vi "Stepper Motor 2.3 Working.vi"() -> ()   [LabVIEW 2017]
uses:
  <vilib>/myRIO/Instrument Drivers/Onboard IO/DIO/typedefs/DIO Reference.ctl
  <vilib>/myRIO/Common/Instrument Driver Framework/Utilities/typedefs/myRIO Generic Hardware Reference.ctl
  <vilib>/myRIO/Common/Instrument Driver Framework/Utilities/typedefs/Hardware Version Enum.ctl
  <vilib>/myRIO/Common/Instrument Driver Framework/Utilities/typedefs/myRIO v1.0 Reference.ctl
  <vilib>/myRIO/Common/Instrument Driver Framework/Utilities/typedefs/Generic FPGA Reference.ctl
  <vilib>/myRIO/Common/Instrument Driver Framework/myRIO v1.0/DIO/typedefs/DIO Channels List.ctl
  <vilib>/myRIO/Common/Instrument Driver Framework/myRIO v1.0/DIO/typedefs/DIO Channels Enum.ctl
  <vilib>/userdefined/High Color/nirio_resource_hc.ctl
  <vilib>/myRIO/Common/Instrument Driver Framework/Utilities/vis/Is FPGA Ref Available.vi
  <vilib>/myRIO/Common/Instrument Driver Framework/myRIO v1.0/DIO/vis/myRIO v1.1 Open DIO.vi
  <vilib>/myRIO/Instrument Drivers/Onboard IO/DIO/vis/Write.vi
  <vilib>/myRIO/Common/Instrument Driver Framework/Utilities/vis/Validate Channels.vi
  <vilib>/myRIO/Common/Instrument Driver Framework/myRIO v1.0/DIO/vis/myRIO v1.0 Reserve DIO.vi
  <vilib>/myRIO/Common/Instrument Driver Framework/myRIO v1.0/Resource Manager/vis/myRIO v1.0 Reserve Channel List.vi
  <vilib>/myRIO/Common/Instrument Driver Framework/myRIO v1.0/DIO/vis/myRIO v1.0 Build MUX Configuration DIO.vi
  <vilib>/myRIO/Common/Instrument Driver Framework/myRIO v1.0/Resource Manager/vis/myRIO v1.0 Reserve Channel.vi
  <vilib>/myRIO/Common/Instrument Driver Framework/myRIO v1.0/Resource Manager/vis/myRIO v1.0 Unreserve Channel.vi
  <vilib>/myRIO/Common/Instrument Driver Framework/myRIO v1.0/Resource Manager/vis/myRIO v1.0 Create Configuration List.vi
  <vilib>/myRIO/Common/Instrument Driver Framework/myRIO v1.0/Resource Manager/vis/myRIO v1.0 Build Mutex Name.vi
  <vilib>/Utility/VariantDataType/GetNumericInfo.vi
  <vilib>/Utility/error.llb/Error Cluster From Error Code.vi
  <vilib>/myRIO/Common/Instrument Driver Framework/myRIO v1.0/myRIO v1.1 Open.vi
  <vilib>/myRIO/Common/Instrument Driver Framework/Utilities/vis/IO Manager.vi
  <vilib>/myRIO/Common/Instrument Driver Framework/Utilities/vis/Configuration Manager.vi
  <vilib>/myRIO/Common/Instrument Driver Framework/myRIO v1.0/Resource Manager/vis/myRIO v1.0 Configure IO.vi
  <vilib>/myRIO/Common/Instrument Driver Framework/myRIO v1.0/myRIO v1.0 Close.vi
  <vilib>/myRIO/Common/Instrument Driver Framework/myRIO v1.0/DIO/vis/myRIO v1.0 Write DIO.vi
  <vilib>/myRIO/Express VI/Onboard Devices/LED/LED Express VI.xnode
  <vilib>/myRIO/Instrument Drivers/Onboard IO/DIO/vis/myRIO DIO Open.xnode
  <vilib>/myRIO/Express VI/Onboard IO/DO/DO Express VI.xnode
  <vilib>/myRIO/Instrument Drivers/Onboard IO/DIO/DIO.lvlib
panel:
  in  "y (inches)":dbl
  out "current pps d":dbl
  out "loop num d":i32
  out "nc":dbl format="%.2f"
  out "current pps c":dbl
  out "loop num c":i32
  out "na":dbl format="%.2f"
  out "current pps a":dbl
  out "loop num a":i32
  in  "Dir":bool=TRUE
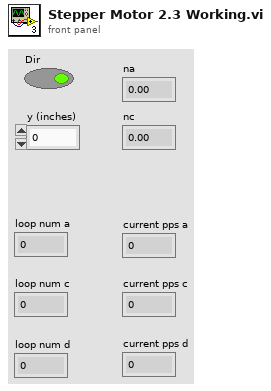
[diagram p1: front panel]
types:
  T1 = typedef "DIO.lvlib/DIO Reference.ctl" = cluster{"myRIO Reference":T2, "DIO Channels List":T6}
  T2 = typedef "myRIO Generic Hardware Reference.ctl" = cluster{"myRIO Model":T3, "myRIO Hardware Reference":T4}
  T3 = typedef "Hardware Version Enum.ctl" = enum16{"Unknown", "myRIO-1900", "myRIO-1950", "roboRIO", "NI ELVIS RIO CM"}
  T4 = typedef "myRIO v1.0 Reference.ctl" = cluster{"Generic FPGA Reference":T5, "Allow multiple opens":bool}
  T5 = typedef "Generic FPGA Reference.ctl" = refnum<k20>
  T6 = typedef "DIO Channels List.ctl" = T7[]
  T7 = typedef "DIO Channels Enum.ctl" = enum16{"Not Connected", "C/DIO0", "C/DIO1", "C/DIO2", "C/DIO3", "C/DIO4", "C/DIO5", "C/DIO6", "C/DIO7", "A/DIO0", "A/DIO1", "A/DIO2", "A/DIO3", "A/DIO4", "A/DIO5", "A/DIO6", "A/DIO7", "A/DIO8", "A/DIO9", "A/DIO10", "A/DIO11", "A/DIO12", "A/DIO13", "A/DIO14", "A/DIO15", "B/DIO0", "B/DIO1", "B/DIO2", "B/DIO3", "B/DIO4", "B/DIO5", "B/DIO6", "B/DIO7", "B/DIO8", "B/DIO9", "B/DIO10", "B/DIO11", "B/DIO12", "B/DIO13", "B/DIO14", "B/DIO15", "LED0", "LED1", "LED2", "LED3", "Button0", "DIO/DIO0", "DIO/DIO1", "DIO/DIO2", "DIO/DIO3", "DIO/DIO4", "DIO/DIO5", "DIO/DIO6", "DIO/DIO7", "DIO/DIO8", "DIO/DIO9", "SPI/CS0", "SPI/CS1", "SPI/CS2", "SPI/CS3", "LED RADIO (Green)", "LED RADIO (Red)", "LED COMM (Green)", "LED COMM (Red)", "LED MODE (Green)", "LED MODE (Red)"}
  T8 = typedef "nirio_resource_hc.ctl" = tag
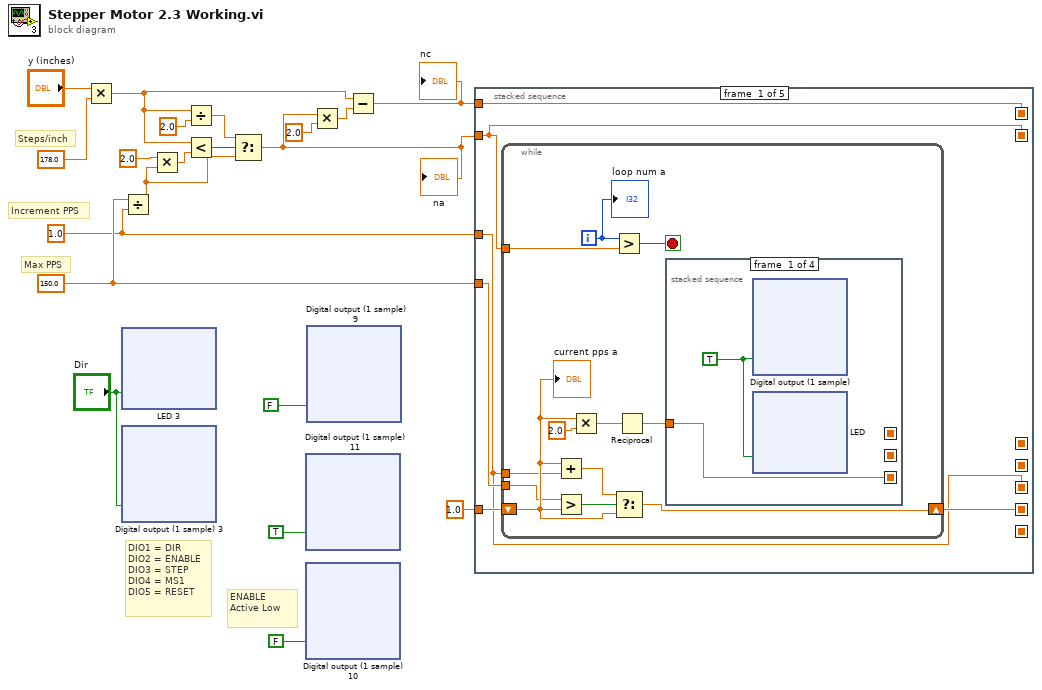
[diagram p0: block diagram]
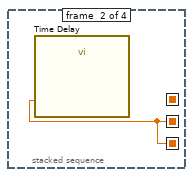
[diagram p2: hidden frame]
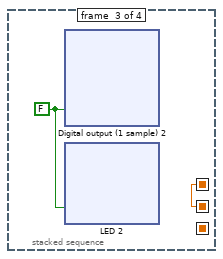
[diagram p3: hidden frame]
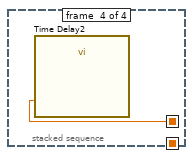
[diagram p4: hidden frame]
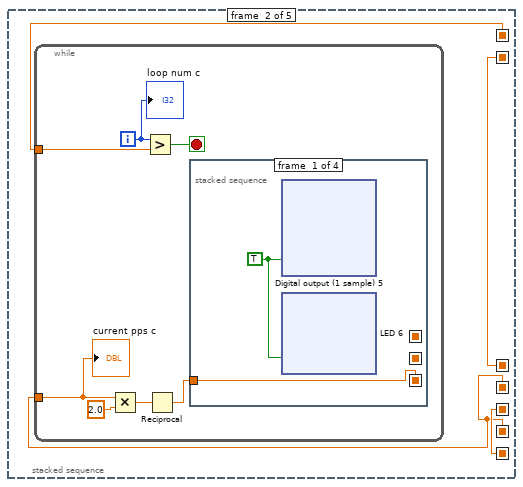
[diagram p5: hidden frame]
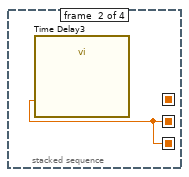
[diagram p6: hidden frame]
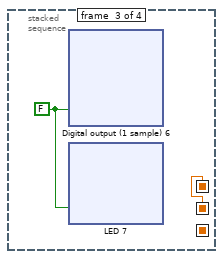
[diagram p7: hidden frame]
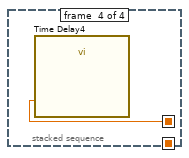
[diagram p8: hidden frame]
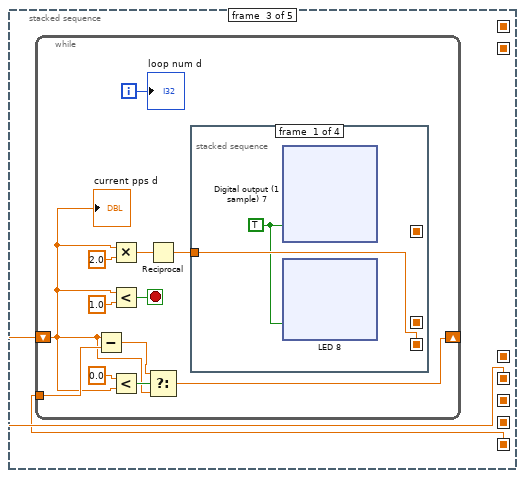
[diagram p9: hidden frame]
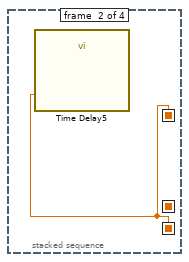
[diagram p10: hidden frame]
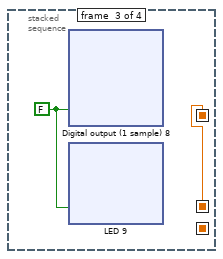
[diagram p11: hidden frame]
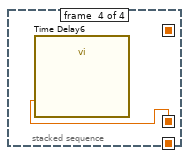
[diagram p12: hidden frame]
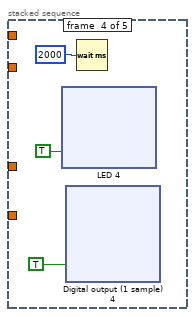
[diagram p13: hidden frame]
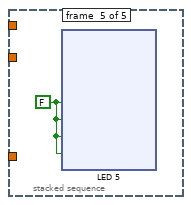
[diagram p14: hidden frame]
diagram:
  w15 = 1.0 ("increment pps")
  w16 = 150.0 ("max pps")
  # "Increment PPS"
  # "Steps/inch"
  # "Max PPS"
  # "ENABLE\nActive Low"
  # "DIO1 = DIR\nDIO2 = ENABLE\nDIO3 = STEP\nDIO4 = MS1\nDIO5 = RESET"
  n1 = Multiply(x="y (inches)", y=178.0 ("steps/in")) -> (x*y=w7:dbl)
  n2 = xnode "LED 3"("LED0"="Dir") -> ()  [unwired: 1 in, 1 out]
  n3 = xnode "Digital output (1 sample) 3"("DIR (A/DIO1 (Pin 13))"="Dir") -> ()  [unwired: 1 in, 1 out]
  n4 = Divide(x=w16, y=w15) -> (x/y=w4:dbl)
  n5 = Multiply(x=2.0 ("y"), y=w4) -> (x*y=w14:dbl)
  n6 = Divide(x=w7, y=2.0) -> (x/y=w11:dbl)
  n7 = Less?(x=w7, y=w14) -> (x < y?=w13:bool)
  n8 = Select(t=w11, s=w13, f=w4) -> (s? t:f=w8:dbl)
  "na" <- w8
  n9 = xnode "Digital output (1 sample) 11"("A/DIO5 (Pin 21)"=TRUE) -> ()  [unwired: 1 in, 1 out]
  n10 = xnode "Digital output (1 sample) 10"("A/DIO2 (Pin 15)"=FALSE) -> ()  [unwired: 1 in, 1 out]
  n11 = xnode "Digital output (1 sample) 9"("A/DIO4 (Pin 19)"=FALSE) -> ()  [unwired: 1 in, 1 out]
  n12 = Multiply(x=w8, y=2.0) -> (x*y=w10:dbl)
  n13 = Subtract(x=w7, y=w10) -> (x-y=w6:dbl)
  "nc" <- w6
  n14 = stacked-sequence {
    seq-local: [w24 _ _ _ _] -> [_ w185 _ _ _]
    seq-local: [w23 _ _ _ _] -> [_ w186 _ _ _]
    seq-local: [w22 _ _ _ _] -> [_ w188 _ _ _]
    seq-local: [w21 _ _ _ _] -> [_ w187 _ _ _]
    seq-local: [_ w188 _ _ _] -> [_ _ w342 _ _]
    seq-local: [_ w187 _ _ _] -> [_ _ _ _ _]
    seq-local: [_ w186 _ _ _] -> [_ _ w343 _ _]
    tunnel: w16 -> [w26 _ _ _ _]
    tunnel: w15 -> [w22 _ _ _ _]
    tunnel: 1.0 ("starting pps") -> [w25 _ _ _ _]
    tunnel: w8 -> [w21 _ _ _ _]
    tunnel: w6 -> [w24 _ _ _ _]
    frame #0 {
      n15 = while {
        shift-right: [w33] -> w23
        shift-left: w25 -> [w32]
        tunnel: w26 -> [w31]
        tunnel: w22 -> [w30]
        tunnel: w21 -> [w28]
        i -> [w27]
        stop <- w29 stop-if-true
        n16 = Add(x=w32, y=w30) -> (x+y=w34:dbl)
        n17 = Greater?(x=w31, y=w32) -> (0:w35:bool)
        n18 = Multiply(x=w32, y=2.0) -> (x*y=w38:dbl)
        n19 = Greater?(x=w27, y=w28) -> (0:w29:bool)
        n20 = Select(t=w34, s=w35, f=w32) -> (s? t:f=w33:dbl)
        n21 = Reciprocal(x=w38) -> (1/x=w36:dbl)
        n22 = stacked-sequence {
          seq-local: [w40 _ _ _] -> [_ w111 _ _]
          seq-local: [_ w111 _ _] -> [_ _ w113 _]
          seq-local: [_ _ w113 _] -> [_ _ _ w184]
          tunnel: w36 -> [w40 _ _ _]
          frame #0 {
            w39 = TRUE
            n23 = xnode "Digital output (1 sample)"("A/DIO3 (Pin 17)"=w39) -> ()  [unwired: 1 in, 1 out]
            n24 = xnode "LED"("LED1"=w39) -> ()  [unwired: 1 in, 1 out]
          }
          frame #1 {
            n25 = call "Time Delay"("Delay Time (s)"=w111) -> ()  [unwired: 10 in, 1 out]
          }
          frame #2 {
            w112 = FALSE
            n26 = xnode "Digital output (1 sample) 2"("A/DIO3 (Pin 17)"=w112) -> ()  [unwired: 1 in, 1 out]
            n27 = xnode "LED 2"("LED1"=w112) -> ()  [unwired: 1 in, 1 out]
          }
          frame #3 {
            n28 = call "Time Delay2"("Delay Time (s)"=w184) -> ()  [unwired: 10 in, 1 out]
          }
        }
        "current pps a" <- w32
        "loop num a" <- w27
      }
    }
    frame #1 {
      n29 = while {
        tunnel: w185 -> [w190]
        tunnel: w186 -> [w192]
        i -> [w189]
        stop <- w191 stop-if-true
        n30 = Multiply(x=w192, y=2.0) -> (x*y=w195:dbl)
        n31 = Greater?(x=w189, y=w190) -> (0:w191:bool)
        n32 = Reciprocal(x=w195) -> (1/x=w193:dbl)
        n33 = stacked-sequence {
          seq-local: [w197 _ _ _] -> [_ w268 _ _]
          seq-local: [_ w268 _ _] -> [_ _ w270 _]
          seq-local: [_ _ w270 _] -> [_ _ _ w341]
          tunnel: w193 -> [w197 _ _ _]
          frame #0 {
            w196 = TRUE
            n34 = xnode "Digital output (1 sample) 5"("A/DIO3 (Pin 17)"=w196) -> ()  [unwired: 1 in, 1 out]
            n35 = xnode "LED 6"("LED1"=w196) -> ()  [unwired: 1 in, 1 out]
          }
          frame #1 {
            n36 = call "Time Delay3"("Delay Time (s)"=w268) -> ()  [unwired: 10 in, 1 out]
          }
          frame #2 {
            w269 = FALSE
            n37 = xnode "Digital output (1 sample) 6"("A/DIO3 (Pin 17)"=w269) -> ()  [unwired: 1 in, 1 out]
            n38 = xnode "LED 7"("LED1"=w269) -> ()  [unwired: 1 in, 1 out]
          }
          frame #3 {
            n39 = call "Time Delay4"("Delay Time (s)"=w341) -> ()  [unwired: 10 in, 1 out]
          }
        }
        "current pps c" <- w192
        "loop num c" <- w189
      }
    }
    frame #2 {
      n40 = while {
        shift-right: [w347] -> _
        shift-left: w343 -> [w345]
        tunnel: w342 -> [w349]
        i -> [w346]
        stop <- w355 stop-if-true
        n41 = Subtract(x=w345, y=w349) -> (x-y=w351:dbl)
        n42 = Multiply(x=w345, y=2.0) -> (x*y=w354:dbl)
        n43 = Less?(x=w345, y=1.0) -> (x < y?=w355:bool)
        n44 = Less?(x=0.0, y=w345) -> (x < y?=w352:bool)
        n45 = Reciprocal(x=w354) -> (1/x=w350:dbl)
        n46 = Select(t=w351, s=w352, f=w345) -> (s? t:f=w347:dbl)
        n47 = stacked-sequence {
          seq-local: [w357 _ _ _] -> [_ w428 _ _]
          seq-local: [_ w428 _ _] -> [_ _ w430 _]
          seq-local: [_ _ w430 _] -> [_ _ _ w501]
          tunnel: w350 -> [w357 _ _ _]
          frame #0 {
            w356 = TRUE
            n48 = xnode "Digital output (1 sample) 7"("A/DIO3 (Pin 17)"=w356) -> ()  [unwired: 1 in, 1 out]
            n49 = xnode "LED 8"("LED1"=w356) -> ()  [unwired: 1 in, 1 out]
          }
          frame #1 {
            n50 = call "Time Delay5"("Delay Time (s)"=w428) -> ()  [unwired: 10 in, 1 out]
          }
          frame #2 {
            w429 = FALSE
            n51 = xnode "Digital output (1 sample) 8"("A/DIO3 (Pin 17)"=w429) -> ()  [unwired: 1 in, 1 out]
            n52 = xnode "LED 9"("LED1"=w429) -> ()  [unwired: 1 in, 1 out]
          }
          frame #3 {
            n53 = call "Time Delay6"("Delay Time (s)"=w501) -> ()  [unwired: 10 in, 1 out]
          }
        }
        "loop num d" <- w346
        "current pps d" <- w345
      }
    }
    frame #3 {
      n54 = xnode "LED 4"("LED2"=TRUE) -> ()  [unwired: 1 in, 1 out]
      n55 = xnode "Digital output (1 sample) 4"("A/DIO2 (Pin 15)"=TRUE) -> ()  [unwired: 1 in, 1 out]
      n56 = Wait (ms)(milliseconds to wait=u32 2000) -> ()  [unwired: 1 out]
    }
    frame #4 {
      w575 = FALSE
      n57 = xnode "LED 5"("LED0"=w575, "LED1"=w575, "LED2"=w575, "LED3"=w575) -> ()  [unwired: 1 in, 1 out]
    }
  }
